vi "calculate #pixels.vi"(8 "error in (no error)":errorcluster, 11 "Simulated Camera in":refnum<class "Sim_CCD.lvclass">) -> (0 "error out":errorcluster, 2 "#pixels":dbl, 3 "Simulated Camera out":refnum<class "Sim_CCD.lvclass">)   [LabVIEW 2018, in "Sim_CCD.lvclass"]
uses:
  Sim_CCD.lvclass
  Sim_CCD.lvclass/Sim_CCD.ctl
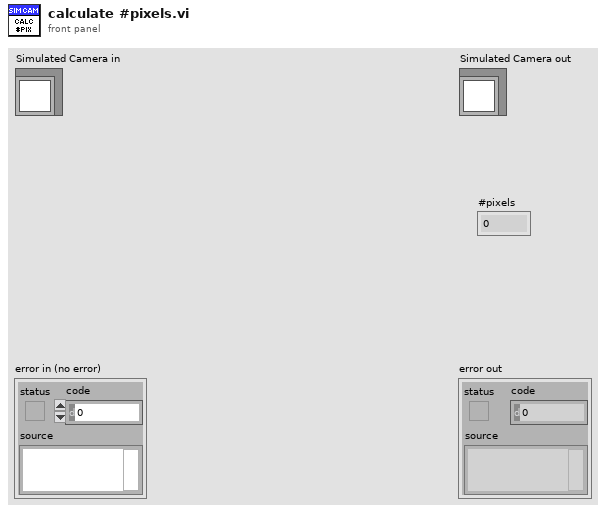
[diagram p1: front panel]
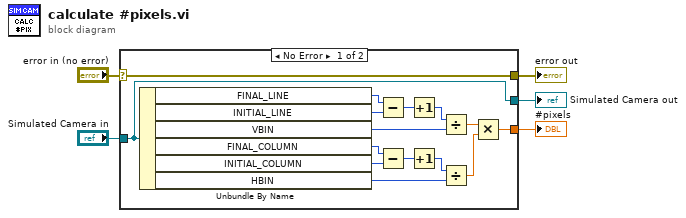
[diagram p0: block diagram]
diagram:
  n1 = case shown="No Error" "error in (no error)" {
    selector: "error in (no error)" -> [w20 w22]
    tunnel: [w20 w22] -> w4
    tunnel: [w6 w21] -> w2
    tunnel: "Simulated Camera in" -> [w6 w21]
    tunnel: [w13 _] -> w1
    frame No Error {
      n2 = Unbundle By Name(w6) -> ("FINAL_LINE"=w12:u16, "INITIAL_LINE"=w11:u16, "VBIN"=w8:u16, "FINAL_COLUMN"=w10:u16, "INITIAL_COLUMN"=w9:u16, "HBIN"=w7:u16)
      n3 = Subtract(x=w12, y=w11) -> (x-y=w19:u16)
      n4 = Subtract(x=w10, y=w9) -> (x-y=w18:u16)
      n5 = Increment(x=w19) -> (x+1=w17:u16)
      n6 = Increment(x=w18) -> (x+1=w16:u16)
      n7 = Divide(x=w17, y=w8) -> (x/y=w15:dbl)
      n8 = Divide(x=w16, y=w7) -> (x/y=w14:dbl)
      n9 = Multiply(x=w15, y=w14) -> (x*y=w13:dbl)
    }
    frame Error {
    }
  }
  "error out" <- w4
  "Simulated Camera out" <- w2
  "#pixels" <- w1
